vi "Set control with signaling_tab.vi"(8 "Value (Signaling)":variant=variant(bool TRUE), 9 "Control Name":string="New/Stop", 10 "VI Name":string="NML Data Acquisition-New.vi", 11 "machine name":string) -> (0 "error out":errorcluster)   [LabVIEW 2020]
panel:
  in  "Tab Control":enum32{"Control", "Statistics"}(tab)
  out "Array":string[](array[string])
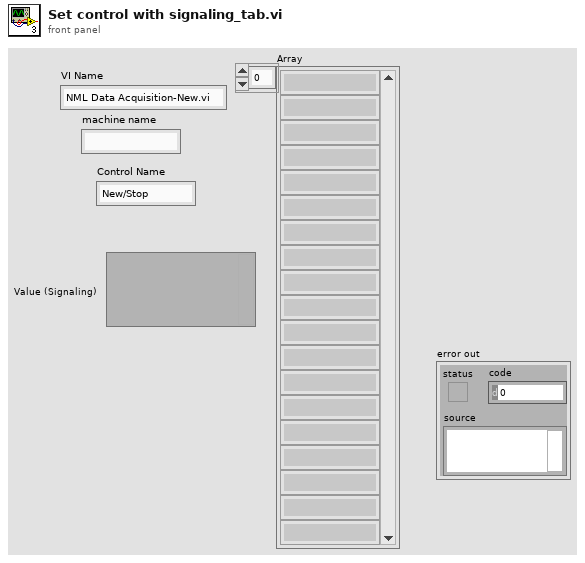
[diagram p1: front panel]
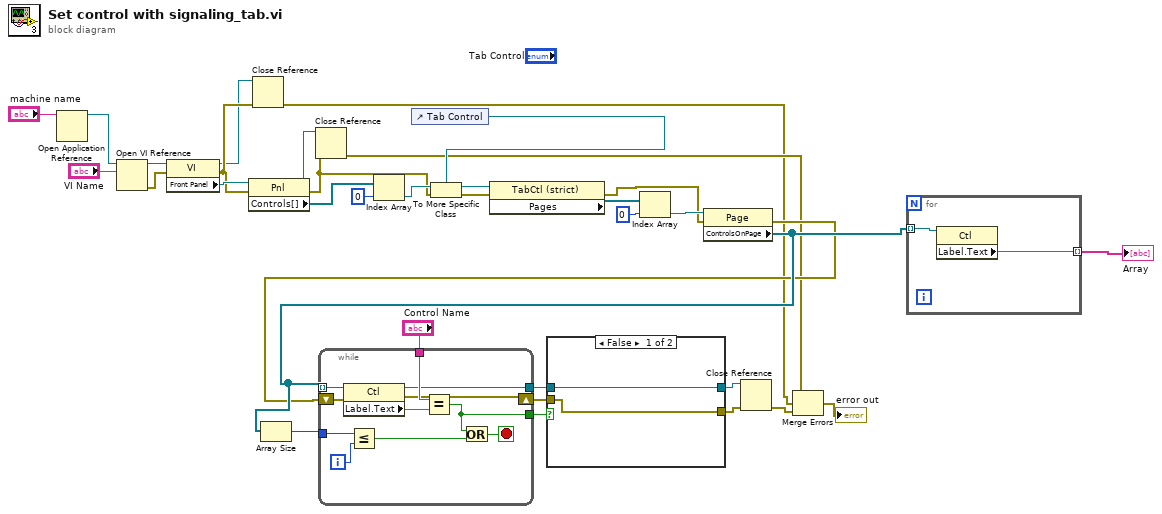
[diagram p0: block diagram]
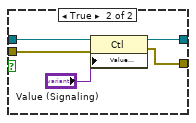
[diagram p2: hidden frame]
diagram:
  n1 = Open Application Reference(11:"machine name") -> (3:w30:refnum<vi>)  [unwired: 3 in, 1 out]
  n2 = Open VI Reference(application reference (local)=w30, vi path="VI Name") -> (vi reference=w34:refnum<vi>, error out=w32:errorcluster)  [unwired: 4 in]
  n3 = property class="VI"(reference=w34, error in=w32) -> (reference out=w2:refnum<vi>, error out=w4:errorcluster, "Front Panel"=w33:refnum<vi>)
  n4 = property class="Pnl"(reference=w33, error in=w4) -> (reference out=w1:refnum<vi>, error out=w7:errorcluster, "Controls[]"=w27:refnum<vi>[])
  n5 = Close Reference(reference=w2, error in (no error)=w4) -> (error out=w3:errorcluster)
  n6 = Close Reference(reference=w1, error in (no error)=w7) -> (error out=w6:errorcluster)
  n7 = Index Array(array=w27, index=0) -> (element=w21:refnum<vi>)
  n8 = control-ref of="Tab Control"() -> (w20:refnum<vi>)
  n9 = To More Specific Class(target class=w20, reference=w21, error in=w7) -> (specific class reference=w25:refnum<vi>, error out=w8:errorcluster)
  n10 = property class="TabCtl (strict)"(reference=w25, error in=w8) -> (error out=w5:errorcluster, "Pages"=w23:refnum<vi>[])  [unwired: 1 out]
  n11 = Index Array(array=w23, index=0) -> (element=w22:refnum<vi>)
  n12 = property class="Page"(reference=w22, error in=w5) -> (error out=w9:errorcluster, "ControlsOnPage"=w10:refnum<vi>[])  [unwired: 1 out]
  n13 = Array Size(array=w10) -> (size(s)=w19:i32)
  n14 = while {
    tunnel: w10 -> [w43] mode=indexing
    tunnel: w19 -> [w44]
    tunnel: "Control Name" -> [w41]
    tunnel: [w38] -> w16
    tunnel: [w37] -> w17
    shift-right: [w35] -> w13
    shift-left: w9 -> [w36]
    i -> [w45]
    stop <- w40 stop-if-true
    n15 = property class="Ctl"(reference=w43, error in=w36) -> (reference out=w38:refnum<vi>, error out=w35:errorcluster, "Label.Text"=w42:string)
    n16 = Less Or Equal?(x=w44, y=w45) -> (x <= y?=w39:bool)
    n17 = Equal?(x=w41, y=w42) -> (x = y?=w37:bool)
    n18 = Or(x=w37, y=w39) -> (x .or. y?=w40:bool)
  }
  n19 = case shown="False" w17 {
    tunnel: w16 -> [w46 w52]
    tunnel: [w46 w51] -> w15
    tunnel: [w47 w50] -> w14
    tunnel: w13 -> [w47 w49]
    frame False {
    }
    frame True {
      n20 = property class="Ctl"(reference=w52, error in=w49, "Value (Signaling)"="Value (Signaling)") -> (reference out=w51:refnum<vi>, error out=w50:errorcluster)
    }
  }
  n21 = Close Reference(reference=w15, error in (no error)=w14) -> (error out=w12:errorcluster)
  n22 = Merge Errors(w6, w3, w12) -> (→"error out":errorcluster)
  n23 = for {
    tunnel: w10 -> [w54] mode=indexing
    tunnel: [w53] -> w28 mode=indexing
    n24 = property class="Ctl"(reference=w54) -> ("Label.Text"=w53:string)  [unwired: 1 in, 2 out]
  }
  "Array" <- w28
